vi "写入零件加工（抽象）.lvclass.vi"(8 "error in (no error)":errorcluster caption="错误输入（无错误）", 10 "零件加工（抽象）.lvclass":refnum<class "零件加工（抽象）.lvclass">, 11 "零件加工流程输入":refnum<class "零件加工流程.lvclass">) -> (0 "error out":errorcluster caption="错误输出", 3 "零件加工流程输出":refnum<class "零件加工流程.lvclass">)   [LabVIEW 2013, in "零件加工流程.lvclass"]
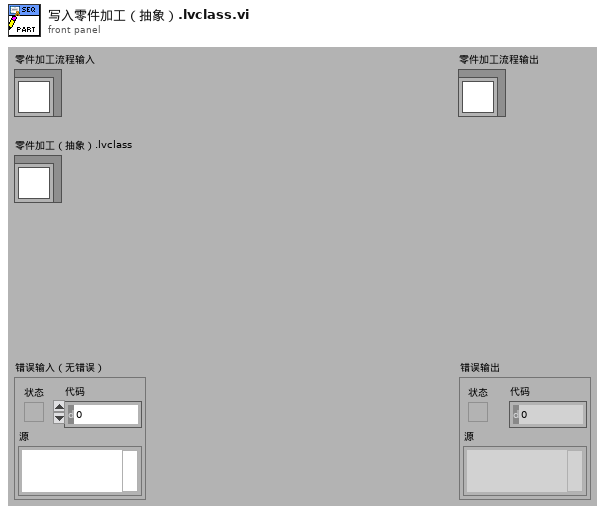
[diagram p1: front panel]
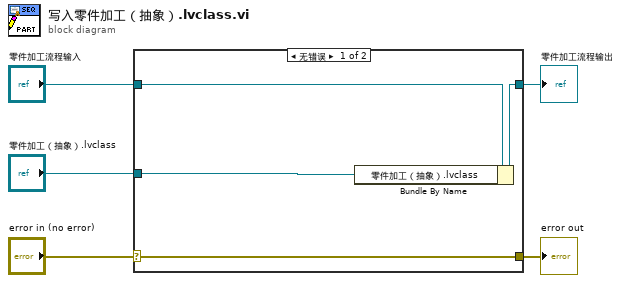
[diagram p0: block diagram]
diagram:
  n1 = case shown="无错误" "error in (no error)" {
    selector: "error in (no error)" -> [w9 w10]
    tunnel: [w9 w10] -> w4
    tunnel: [w7 w11] -> w2
    tunnel: "零件加工流程输入" -> [w8 w11]
    tunnel: "零件加工（抽象）.lvclass" -> [w6 _]
    frame No Error {
      n2 = Bundle By Name(cluster=w8, "零件加工（抽象）.lvclass"=w6) -> (w7:refnum<class "零件加工流程.lvclass">)
    }
    frame Error {
    }
  }
  "error out" <- w4
  "零件加工流程输出" <- w2
